vi "RegisterConductanceEvent.vi"(8 "error in (no error)":errorcluster, 11 "handle":u64) -> (0 "error out":errorcluster, 3 "Conductance Event":refnum<user-event>)   [LabVIEW 2015, in "ReDeX.lvlib"]
doc: "redex_lv_result redex_lv_register_conductance_event(redex_lv_handle handle,\n redex_lv_event_ref *ref);"
uses:
  ReDeX.lvlib
  C:/ReDeX/ReDeX.dll
panel:
  out "function return":u32(ring)
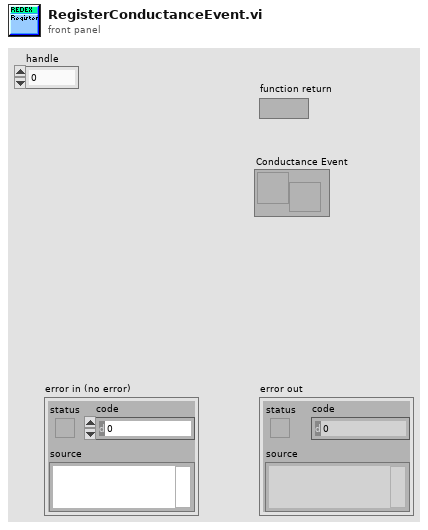
[diagram p1: front panel]
types:
  T1 = cluster{"Testpoint ID":string, "Voltage":dbl, "Current":dbl, "Admittance":dbl}
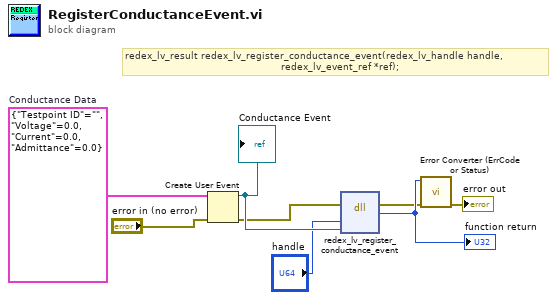
[diagram p0: block diagram]
diagram:
  w5 = T1 {"Testpoint ID"="", "Voltage"=0.0, "Current"=0.0, "Admittance"=0.0}  # Conductance Data
  # "redex_lv_result redex_lv_register_conductance_event(redex_lv_handle handle,\n                                                    redex_lv_event_ref *ref);"
  n1 = Create User Event(user event datatype=w5, error in="error in (no error)") -> (user event=w4:refnum<user-event>, error out=w2:errorcluster)
  "Conductance Event" <- w4
  n2 = dll-call lib="C:/ReDeX/ReDeX.dll" fn="redex_lv_register_conductance_event"(error in=w2, "handle"="handle", "ref"=w4) -> (error out=w7:errorcluster, "return type"=w8:u32)  [unwired: 4 in, 1 out]
  "function return" <- w8
  n3 = call "Error Converter (ErrCode or Status).vi"("error in (no error)"=w7, "error code"=w8) -> ("error out"=→"error out":errorcluster)  [unwired: 9 in]
